vi "GetUID.vi"(6 "error in":errorcluster, 9 "GObject in":refnum<class "GObject.lvclass">) -> (0 "error out":errorcluster, 3 "GObject out":refnum<class "GObject.lvclass">, 4 "UID":i32)   [LabVIEW 2014, in "GObject.lvclass"]
uses:
  GObject.lvclass
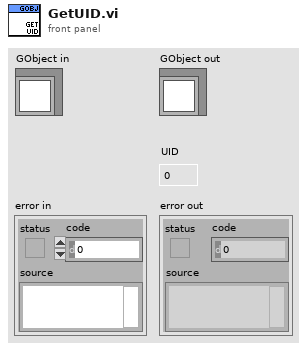
[diagram p1: front panel]
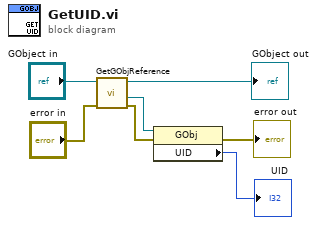
[diagram p0: block diagram]
diagram:
  n1 = call "GetGObjReference.vi"("error in"="error in", "GObject in"="GObject in") -> ("error out"=w4:errorcluster, "reference out"=w3:refnum<vi>, "GObject out"=→"GObject out":refnum<class "GObject.lvclass">)  [unwired: 5 in]
  n2 = property class="GObj"(reference=w3, error in=w4) -> (error out=→"error out":errorcluster, "UID"=→"UID":i32)  [unwired: 1 out]
